vi "Radar_LVDT_updated.vi"(0 "VISA resource name":refnum<visa-resource-name>="COM1", 1 "baud rate":u32=9600, 4 "data bits":u16=8 min=5 max=8 step=1, 5 "parity":u16(ring) items=["None", "Odd", "Even", "Mark", "Space"], 7 "stop bits":u16(ring)=10 items=["1.0"=10, "1.5"=15, "2.0"=20], 9 "XON Character":u8=17 format="%.0x", 14 "XOFF Character":u8=19 format="%.0x", 15 "timeout (ms)":u32=10000, 21 "End read on termination character?":bool=TRUE, 24 "termination char\n(0xA = '\\n' = LF)":u8=10 format="%.0x", 25 "Input\nbuffer size":u32=4096) -> ()   [LabVIEW 2010]
doc: "The Advanced Serial Read and Write example performs a Serial Port Read, a Serial Port Write, or a combination of these actions while setting some advanced serial features like buffer size, termination characters, and XON/XOFF flow control. The user selects the actions (read or write) on the front panel. If both are selected, the VI will write the data first, read the data and then close the VISA session that is opened to the port. \n\nThe parameters set for the serial port must match the parameters of the connected instrument or device. In this example, the bytes to read parameter specifies the number of bytes that the serial port reads. If there were more bytes at the port than the number specified in bytes to read, those bytes would not be read. Also, if you specify to read more bytes than the number of bytes actually read, you might receive a timeout error message.\n\nINSTRUCTIONS:\n1) Select the serial resource and configuration parameters (baud rate, data bits, parity, stop bits, flow control).\n2) Termination character can be enabled and set. Also, set the required input buffer size prior to running the example.\n3) Select the operations to be performed. \n4) Connect the serial port to your device. If no device is available, perform a loopback test by doing one of the following. Short pins 2 and 3 on a RS-232 cable or short pin 4 to pin 8 and pin 5 to pin 9 on a RS-485/422 cable. \n5) Run the VI to see the data read. (The \"read string\" will match the \"string to write\" if a loopback test was performed.)\n\nThis example exposes several advanced features that you may need for your application. Not all applications need all the features shown in this example. The input buffer size is likely an important setting that you want to control in your application. This example expands upon the flow control option for XON and XOFF, allowing the user to choose those control characters. The timeout parameter has been brought to the front panel so a user can specify the time period the VISA Read will wait for the number of bytes to read before timing out. Also, the user has several controls for the termination character, which is discussed later.\n\nNote that you can press the write and read buttons and change the bytes to read parameters on the fly, while the example is running. However, you must stop the example to change the other configuration parameters after the example has started running, and then run again.\n\nSet the I/O buffer size slightly higher the amount of data you expect to receive. This is very important for applications that don't use flow control, as you may lose characters if the receive buffer overflows.\n\nSetting the timeout period ensures that the operation returns with a timeout error if the operation cannot be performed in the specified time period. \n\nSome devices require a termination character in order to identify the end of command strings. Some devices send a termination character to signify the end of data to be read. \n\nThis example shows how you can end the Read operation once a termination character is detected in the buffer and/or append a termination character at the end of the Write data. To enable the Read to end on a termination character, use the VISA Configure Serial Port or use the VISA Properties Serial End Mode for Reads, Termination Character Enable, and Termination Character. To end the Write with a termination character, use the VISA Properties Serial End Mode for Writes, the Send End Enable, and Termination Character. In this example, the same termination character is used for both the Read and the Write. You can specify two different characters for your application, if desired.\n\nYour application may require specific characters for the XON/XOFF Flow Control. You can specify these characters with the VISA Properties Flow Control XOFF Character and Flow Control XON Character. Note that if the standard XON and XOFF characters are used, then decimal 17 and 19 are unavailable for data values. Remember that using flow control and setting an adequate buffer size allow you to prevent buffer overflows."
uses:
  <vilib>/Instr/_visa.llb/VISA Configure Serial Port (Instr).vi
panel:
  in  "Radar2_I Filename":string
  in  "Radar1_I Filename":string
  in  "Radar2_Q Filename":string
  in  "Radar1_Q Filename":string
  in  "LVDT Filename":string
  in  "stop 2":bool
  out "Waveform Graph":dynamicdata(graph)
  out "I/Q channels 2":dynamicdata(graph)
  in  "Save Data":bool
  out "I/Q  Channels 1":dynamicdata(graph)
  in  "t0":timestamp=timestamp(3198752888.296 s since 1904-01-01)
  in  "FFT":i32=256
  in  "stop":bool
  in  "flow control":u16(ring) items=["None"=0, "XON/XOFF"=1, "RTS/CTS"=2, "DTR/DSR"=4]
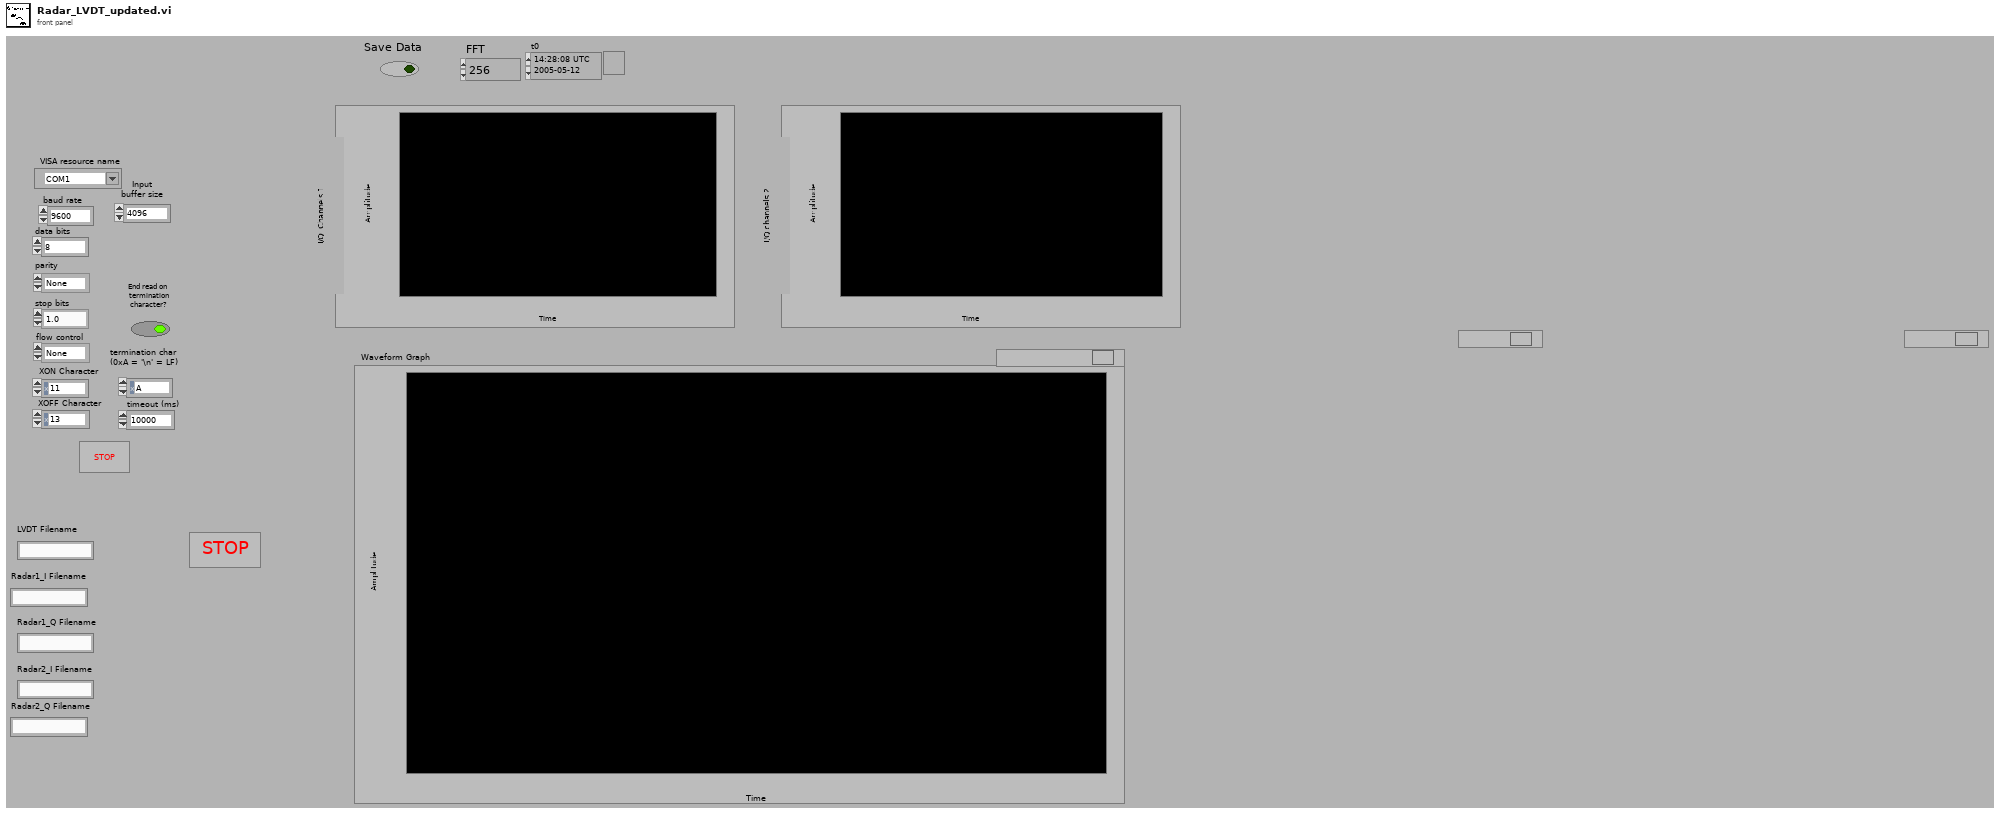
[diagram p1: front panel]
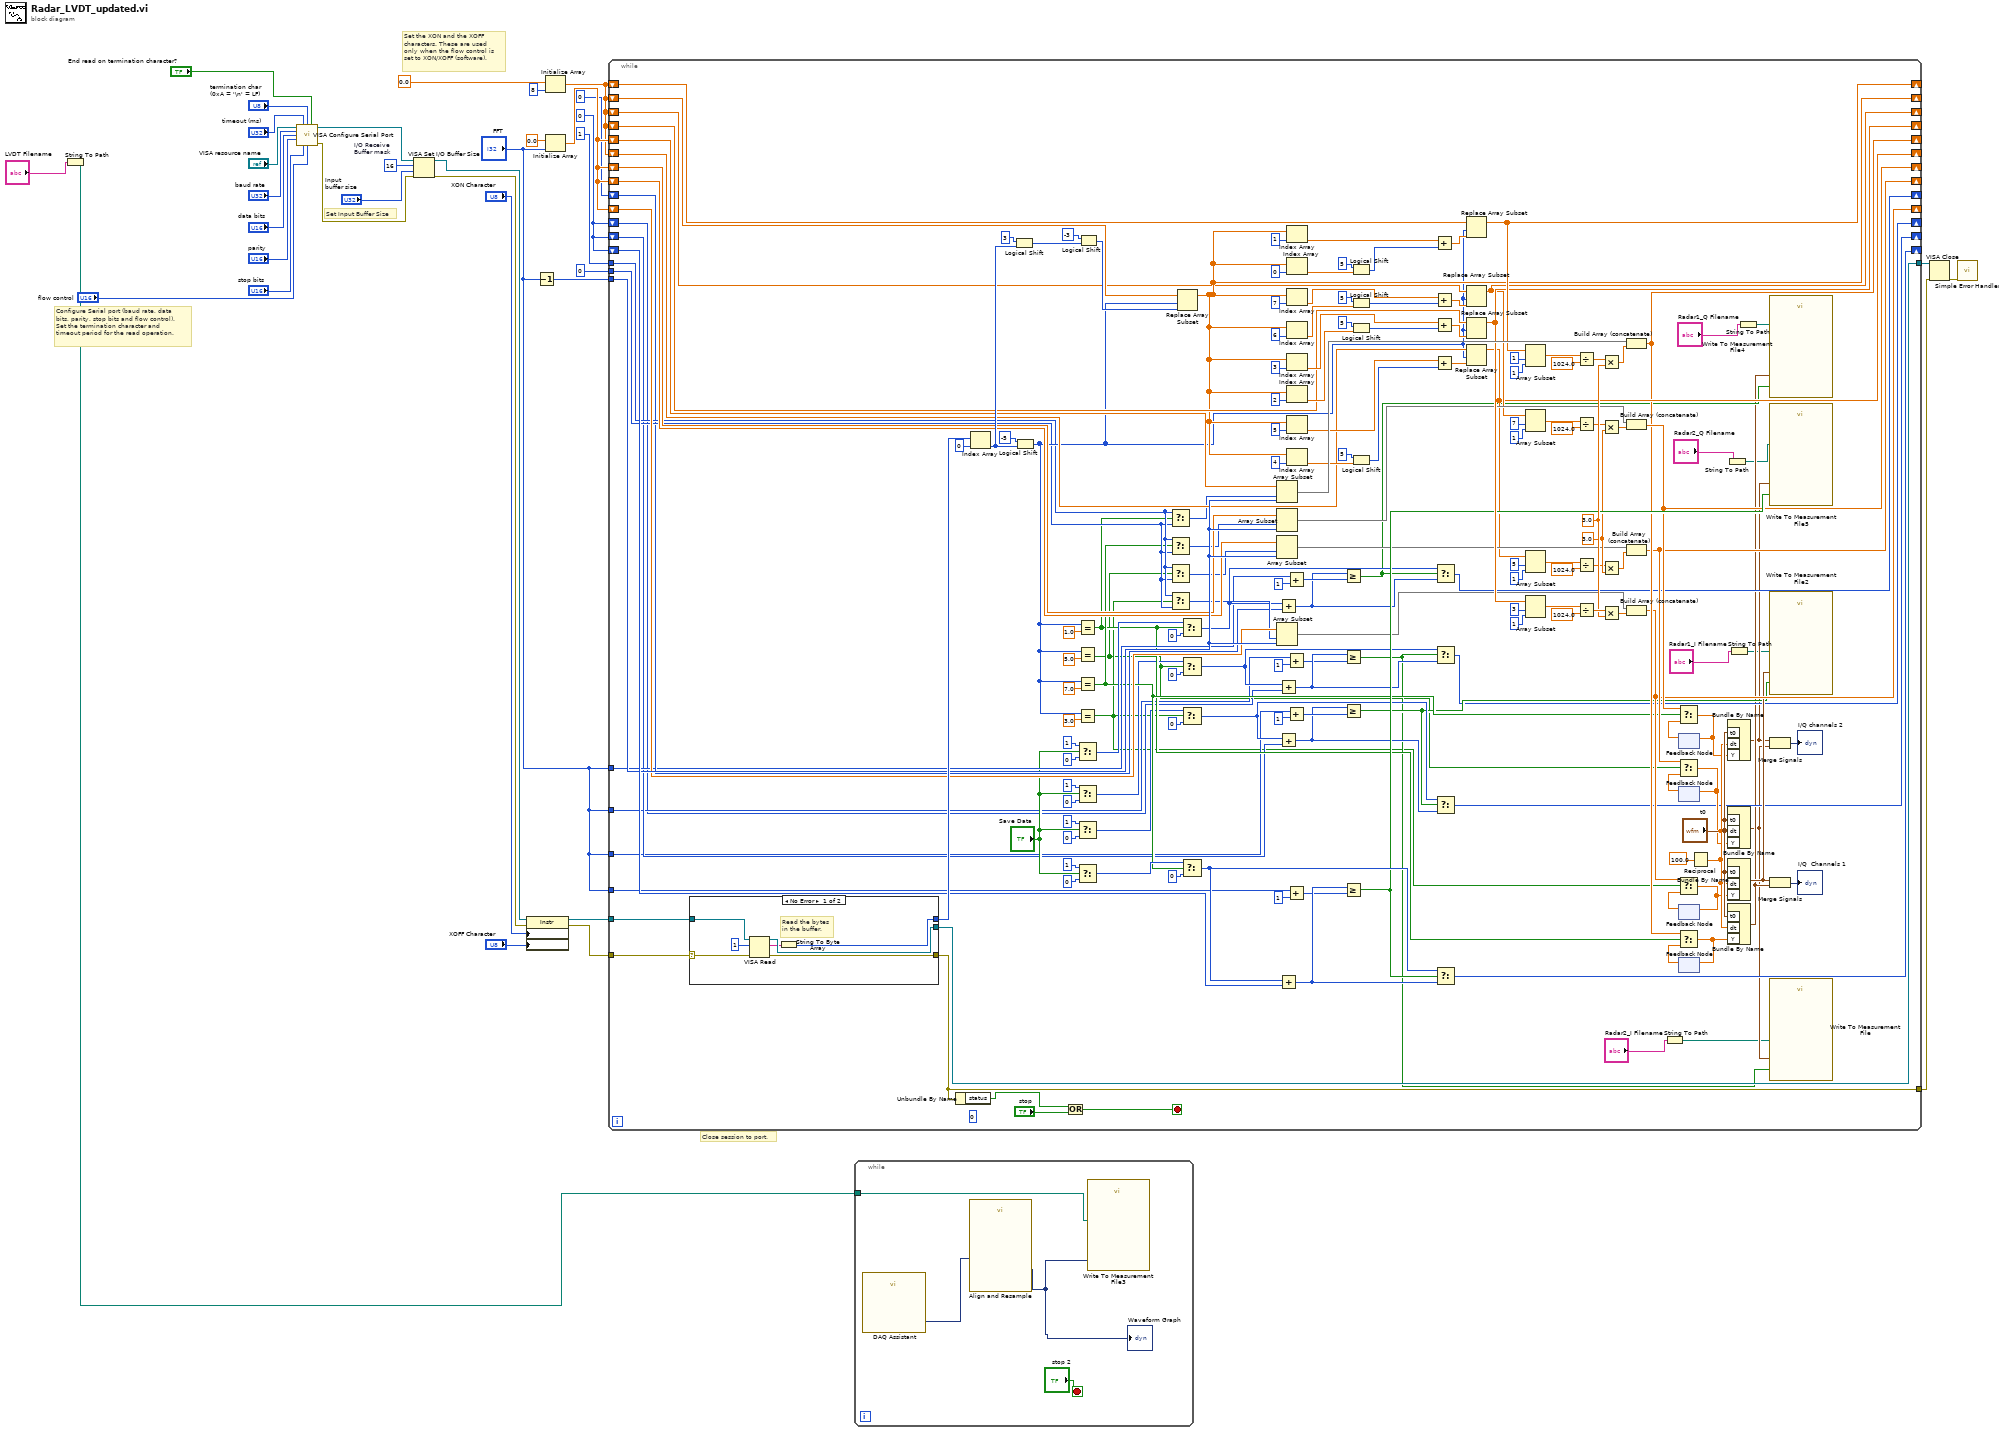
[diagram p0: block diagram]
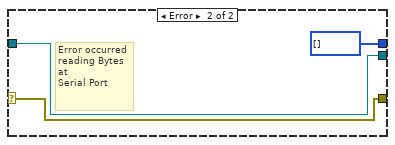
[diagram p2: hidden frame]
diagram:
  w3 = 0
  w28 = u16 16  # I/O Receive Buffer mask
  # "Set the XON and the XOFF\ncharacters. These are used\nonly when the flow control is\nset to XON/XOFF (software)."
  # "Configure Serial port (baud rate, data\nbits, parity, stop bits and flow control).\nSet the termination character and\ntimeout period for the read operation."
  # "Set Input Buffer Size"
  # "Close session to port."
  n1 = String To Path(string="LVDT Filename") -> (path=w1:path)
  n2 = call-poly "VISA Configure Serial Port"("VISA resource name"="VISA resource name", "timeout (10sec)"="timeout (ms)", "termination char\n(0xA = '\\n' = LF)"="termination char\n(0xA = '\\n' = LF)", "Enable Termination\nChar (T)"="End read on termination character?", "baud rate (9600)"="baud rate", "data bits (8)"="data bits", "parity (0:none)"="parity", "stop bits (10: 1 bit)"="stop bits", "flow control (0:none)"="flow control") -> ("VISA resource name out"=w15:refnum<visa-resource-name>, "error out"=w14:errorcluster)  [unwired: 1 in, 4 out]
  n3 = VISA Set I/O Buffer Size(VISA resource name=w15, mask (16)=w28, size (4096)="Input\nbuffer size", error in (no error)=w14) -> (VISA resource name out=w24:refnum<visa-resource-name>, error out=w23:errorcluster)
  n4 = property class="Instr"(reference=w24, error in=w23, "Serial Settings:Flow Control XON Character"="XON Character", "Serial Settings:Flow Control XOFF Character"="XOFF Character") -> (reference out=w18:refnum<visa-resource-name>, error out=w20:errorcluster)
  n5 = Decrement(x="FFT") -> (x-1=w13:i32)
  n6 = Initialize Array(0.0 ("element"), 8 ("dimension size")) -> (w7:dbl[])
  n7 = Initialize Array(0.0 ("element"), "FFT") -> (w8:dbl[])
  n8 = while {
    tunnel: w20 -> [w191]
    tunnel: w18 -> [w192]
    tunnel: [w190] -> w17
    tunnel: [w189] -> w16
    tunnel: w13 -> [w130]
    tunnel: 1 ("index") -> [w99]
    shift-right: [w113] -> _
    shift-left: w8 -> [w131]
    shift-right: [w135] -> _
    shift-left: w7 -> [w206]
    shift-right: [w103] -> _
    shift-left: w8 -> [w105]
    shift-right: [w181] -> _
    shift-left: w7 -> [w183]
    shift-right: [w174] -> _
    shift-left: w7 -> [w177]
    shift-right: [w167] -> _
    shift-left: w3 -> [w170]
    tunnel: "FFT" -> [w164]
    shift-right: [w117] -> _
    shift-left: w8 -> [w128]
    shift-right: [w110] -> _
    shift-left: w8 -> [w126]
    shift-right: [w124] -> _
    shift-left: w7 -> [w125]
    shift-right: [w122] -> _
    shift-left: w7 -> [w123]
    tunnel: 0 ("index") -> [w98]
    shift-right: [w83] -> _
    shift-left: 0 -> [w84]
    tunnel: "FFT" -> [w82]
    tunnel: "FFT" -> [w52]
    tunnel: "FFT" -> [w51]
    shift-right: [w50] -> _
    shift-left: w3 -> [w54]
    shift-right: [w53] -> _
    shift-left: w3 -> [w49]
    stop <- w215 stop-if-true
    w159 = 3.0 ("y")
    (unwired) 0
    w172 = 3.0 ("y")
    n9 = case "Read bytes from port." shown="No Error" w191 {
      selector: w191 -> [w220 w225]
      tunnel: [w222 w225] -> w189
      tunnel: [w223 w226] -> w190
      tunnel: w192 -> [w221 w226]
      tunnel: [w218 u8[] [] ("unsigned byte array")] -> w188
      frame No Error {
        # "Read the bytes\nin the buffer."
        n10 = VISA Read(VISA resource name=w221, byte count=u32 1, error in (no error)=w220) -> (VISA resource name out=w223:refnum<visa-resource-name>, read buffer=w219:string, error out=w222:errorcluster)  [unwired: 1 out]
        n11 = String To Byte Array(string=w219) -> (unsigned byte array=w218:u8[])
      }
      frame Error {
        # "Error occurred \nreading Bytes at \nSerial Port"
      }
    }
    n12 = Unbundle By Name(w189) -> ("status"=w216:bool)
    n13 = Index Array(array=w188, index=0) -> (element=w209:u8)
    n14 = Logical Shift(y=i8 3, x=w209) -> (x << y=w208:u8)
    n15 = Logical Shift(y=i8 -5, x=w209) -> (x << y=w108:u8)
    n16 = Or(x=w216, y="stop") -> (x .or. y?=w215:bool)
    n17 = Select(t=1, s="Save Data", f=0) -> (s? t:f=w86:i32)
    n18 = Select(t=1, s="Save Data", f=0) -> (s? t:f=w60:i32)
    n19 = Select(t=1, s="Save Data", f=0) -> (s? t:f=w62:i32)
    n20 = Select(t=1, s="Save Data", f=0) -> (s? t:f=w81:i32)
    n21 = Equal?(x=w108, y=1.0) -> (x = y?=w77:bool)
    n22 = Equal?(x=w108, y=5.0) -> (x = y?=w47:bool)
    n23 = Equal?(x=w108, y=7.0) -> (x = y?=w78:bool)
    n24 = Equal?(x=w108, y=3.0) -> (x = y?=w48:bool)
    n25 = Logical Shift(y=i8 -3, x=w208) -> (x << y=w205:u8)
    n26 = Select(t=w99, s=w77, f=w98) -> (s? t:f=w101:i32)
    n27 = Select(t=w99, s=w78, f=w98) -> (s? t:f=w100:i32)
    n28 = Select(t=w99, s=w47, f=w98) -> (s? t:f=w97:i32)
    n29 = Select(t=w99, s=w48, f=w98) -> (s? t:f=w102:i32)
    n30 = Replace Array Subset(array=w206, new element=w205, index=w108) -> (w135:dbl[])
    n31 = Select(t=w86, s=w77, f=0) -> (s? t:f=w85:i32)
    n32 = Select(t=w60, s=w47, f=0) -> (s? t:f=w72:i32)
    n33 = Select(t=w62, s=w48, f=0) -> (s? t:f=w61:i32)
    n34 = Select(t=w81, s=w78, f=0) -> (s? t:f=w169:i32)
    n35 = Array Subset(array=w131, index=w101, length=w130) -> (w213:dbl[])
    n36 = Array Subset(array=w128, index=w100, length=w130) -> (w129:dbl[])
    n37 = Array Subset(array=w126, index=w97, length=w130) -> (w127:dbl[])
    n38 = Array Subset(array=w105, index=w102, length=w130) -> (w132:dbl[])
    n39 = Add(x=w85, y=w84) -> (x+y=w90:i32)
    n40 = Add(x=w72, y=w49) -> (x+y=w71:i32)
    n41 = Add(x=w61, y=w54) -> (x+y=w66:i32)
    n42 = Add(x=w169, y=w170) -> (x+y=w168:i32)
    n43 = Add(x=w82, y=1) -> (x+y=w92:i32)
    n44 = Add(x=w51, y=1) -> (x+y=w69:i32)
    n45 = Add(x=w52, y=1) -> (x+y=w68:i32)
    n46 = Add(x=w164, y=1) -> (x+y=w165:i32)
    n47 = Index Array(array=w135, index=1) -> (element=w196:dbl)
    n48 = Index Array(array=w135, index=0) -> (element=w199:dbl)
    n49 = Index Array(array=w135, index=7) -> (element=w146:dbl)
    n50 = Index Array(array=w135, index=6) -> (element=w143:dbl)
    n51 = Index Array(array=w135, index=3) -> (element=w194:dbl)
    n52 = Index Array(array=w135, index=2) -> (element=w197:dbl)
    n53 = Index Array(array=w135, index=5) -> (element=w144:dbl)
    n54 = Index Array(array=w135, index=4) -> (element=w141:dbl)
    n55 = Greater Or Equal?(x=w90, y=w92) -> (x >= y?=w74:bool)
    n56 = Greater Or Equal?(x=w71, y=w69) -> (x >= y?=w55:bool)
    n57 = Greater Or Equal?(x=w66, y=w68) -> (x >= y?=w56:bool)
    n58 = Greater Or Equal?(x=w168, y=w165) -> (x >= y?=w161:bool)
    n59 = Logical Shift(y=i16 5, x=w199) -> (x << y=w195:u32)
    n60 = Logical Shift(y=i16 5, x=w143) -> (x << y=w147:u32)
    n61 = Logical Shift(y=i16 5, x=w197) -> (x << y=w193:u32)
    n62 = Logical Shift(y=i16 5, x=w141) -> (x << y=w145:u32)
    n63 = Add(x=w196, y=w195) -> (x+y=w182:dbl)
    n64 = Add(x=w146, y=w147) -> (x+y=w120:dbl)
    n65 = Add(x=w194, y=w193) -> (x+y=w121:dbl)
    n66 = Add(x=w144, y=w145) -> (x+y=w152:dbl)
    n67 = Select(t=w85, s=w74, f=w90) -> (s? t:f=w83:i32)
    n68 = Select(t=w72, s=w55, f=w71) -> (s? t:f=w53:i32)
    n69 = Select(t=w61, s=w56, f=w66) -> (s? t:f=w50:i32)
    n70 = Select(t=w169, s=w161, f=w168) -> (s? t:f=w167:i32)
    n71 = Replace Array Subset(array=w183, new element=w182, index=w108) -> (w181:dbl[])
    n72 = Replace Array Subset(array=w125, new element=w120, index=w108) -> (w124:dbl[])
    n73 = Replace Array Subset(array=w177, new element=w121, index=w108) -> (w174:dbl[])
    n74 = Replace Array Subset(array=w123, new element=w152, index=w108) -> (w122:dbl[])
    n75 = Array Subset(array=w181, index=1, length=1) -> (w178:dbl[])
    n76 = Array Subset(array=w124, index=7, length=1) -> (w158:dbl[])
    n77 = Array Subset(array=w122, index=5, length=1) -> (w155:dbl[])
    n78 = Array Subset(array=w174, index=3, length=1) -> (w173:dbl[])
    n79 = Divide(x=w178, y=1024.0) -> (x/y=w186:dbl[])
    n80 = Divide(x=w158, y=1024.0) -> (x/y=w151:dbl[])
    n81 = Divide(x=w155, y=1024.0) -> (x/y=w149:dbl[])
    n82 = Divide(x=w173, y=1024.0) -> (x/y=w184:dbl[])
    n83 = Multiply(x=w186, y=w172) -> (x*y=w163:dbl[])
    n84 = Multiply(x=w151, y=w159) -> (x*y=w133:dbl[])
    n85 = Multiply(x=w149, y=w159) -> (x*y=w134:dbl[])
    n86 = Multiply(x=w184, y=w172) -> (x*y=w106:dbl[])
    n87 = Build Array (concatenate)(w213, w163) -> (w113:dbl[])
    n88 = Build Array (concatenate)(w129, w133) -> (w117:dbl[])
    n89 = Build Array (concatenate)(w127, w134) -> (w110:dbl[])
    n90 = Build Array (concatenate)(w132, w106) -> (w103:dbl[])
    n91 = String To Path(string="Radar2_I Filename") -> (path=w36:path)
    n92 = feedback #1() -> (w116:dbl[])  [unwired: 1 out]
    n93 = Select(t=w117, s=w78, f=w116) -> (s? t:f=w96:dbl[])
    n94 = feedback-in #1(w96) -> ()
    n95 = feedback #2() -> (w111:dbl[])  [unwired: 1 out]
    n96 = Select(t=w110, s=w47, f=w111) -> (s? t:f=w95:dbl[])
    n97 = feedback-in #2(w95) -> ()
    n98 = feedback #3() -> (w104:dbl[])  [unwired: 1 out]
    n99 = Select(t=w103, s=w48, f=w104) -> (s? t:f=w94:dbl[])
    n100 = feedback-in #3(w94) -> ()
    n101 = feedback #4() -> (w114:dbl[])  [unwired: 1 out]
    n102 = Select(t=w113, s=w77, f=w114) -> (s? t:f=w93:dbl[])
    n103 = feedback-in #4(w93) -> ()
    n104 = Reciprocal(x=100.0 ("y")) -> (1/x=w107:dbl)
    n105 = String To Path(string="Radar2_Q Filename") -> (path=w40:path)
    n106 = Bundle By Name("t0"="t0", "dt"=w107, "Y"=w96) -> (w44:waveform(dbl))  [unwired: 1 out]
    n107 = Bundle By Name("t0"="t0", "dt"=w107, "Y"=w95) -> (w45:waveform(dbl))  [unwired: 1 out]
    n108 = Bundle By Name("t0"="t0", "dt"=w107, "Y"=w94) -> (w75:waveform(dbl))  [unwired: 1 out]
    n109 = Bundle By Name("t0"="t0", "dt"=w107, "Y"=w93) -> (w46:waveform(dbl))  [unwired: 1 out]
    n110 = String To Path(string="Radar1_I Filename") -> (path=w38:path)
    n111 = String To Path(string="Radar1_Q Filename") -> (path=w42:path)
    n112 = call "Write To Measurement File4"("Signals"=w46, "Enable"=w74, "Filename"=w42) -> ()  [unwired: 14 in, 3 out]
    n113 = call "Write To Measurement File5"("Signals"=w44, "Enable"=w161, "Filename"=w40) -> ()  [unwired: 14 in, 3 out]
    n114 = call "Write To Measurement File2"("Signals"=w75, "Enable"=w56, "Filename"=w38) -> ()  [unwired: 14 in, 3 out]
    n115 = Merge Signals(w44, w45) -> (→"I/Q channels 2":dynamicdata)
    n116 = Merge Signals(w75, w46) -> (→"I/Q  Channels 1":dynamicdata)
    n117 = call "Write To Measurement File"("Signals"=w45, "Enable"=w55, "Filename"=w36) -> ()  [unwired: 14 in, 3 out]
  }
  n118 = while {
    tunnel: w1 -> [w227]
    stop <- "stop 2" stop-if-true
    n119 = call "DAQ Assistant"() -> ("data"=w229:dynamicdata)  [unwired: 16 in, 3 out]
    n120 = call "Align and Resample"("Signals"=w229) -> ("Resampled Signals"=w228:dynamicdata)  [unwired: 8 in, 2 out]
    "Waveform Graph" <- w228
    n121 = call "Write To Measurement File3"("Signals"=w228, "Filename"=w227) -> ()  [unwired: 15 in, 3 out]
  }
  n122 = VISA Close(VISA resource name=w17, error in (no error)=w16) -> (error out=w33:errorcluster)
  n123 = call <vilib>:"Simple Error Handler.vi"("error in (no error)"=w33) -> ()  [unwired: 1 in, 8 out]
